vi "Memory.Array.Set Element Size.vi"(8 "error in (no error)":errorcluster, 10 "size of element":u64 format="%d bytes", 11 "Memory.Array in":refnum<class "Memory.Array.Void.lvclass">) -> (0 "error out":errorcluster, 3 "Memory.Array out":refnum<class "Memory.Array.Void.lvclass">)   [LabVIEW 2016, in "Memory Manager.lvlib" / "Memory.Array.Void.lvclass"]
uses:
  Memory.Array.Void.lvclass
  Memory.Array.Void.lvclass/Memory.Array.Void.ctl
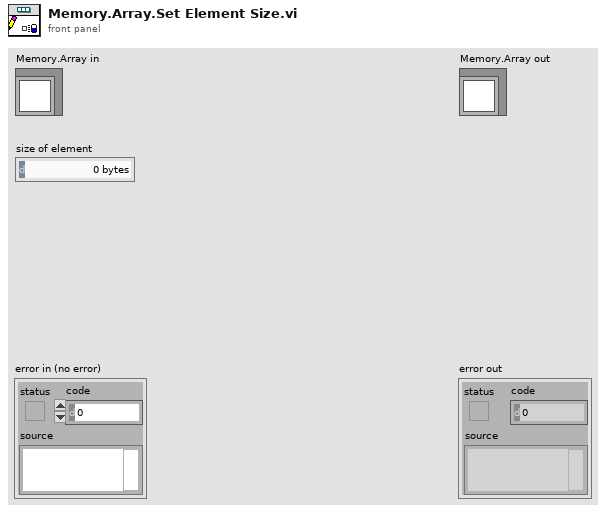
[diagram p1: front panel]
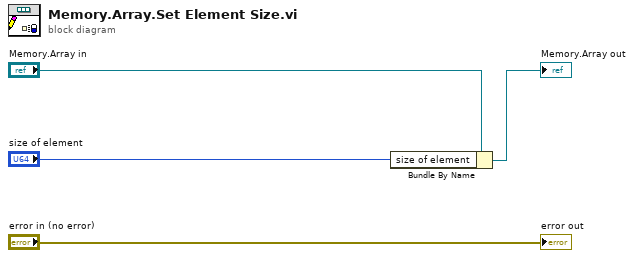
[diagram p0: block diagram]
diagram:
  n1 = Bundle By Name(cluster="Memory.Array in", "size of element"="size of element") -> (→"Memory.Array out":refnum<class "Memory.Array.Void.lvclass">)
  "error out" <- "error in (no error)"
